vi "PH_AxisGUI_6P.PC AbsMove.vi"(0 "i ref in":refnum<vi>, 2 "Axis Selector":T1, 4 "absolute position (units)":dbl, 5 "error in":errorcluster) -> (14 "i ref out":refnum<vi>, 19 "error out":errorcluster)   [LabVIEW 2014]
uses:
  PH_AxisGUI_6P.lvlib
  PH_Common/PH_Motion/PH_Motion.Axis Address.ctl
  PH_AxisGUI_6P.AxisSelector.ctl
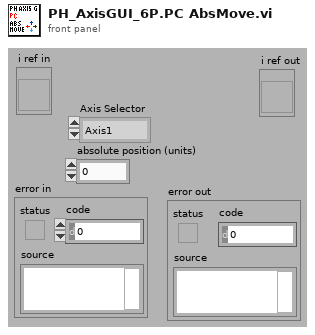
[diagram p1: front panel]
types:
  T1 = typedef "PH_AxisGUI_6P.lvlib/PH_AxisGUI_6P.AxisSelector.ctl" = enum16{"Axis1", "Axis2", "None"}
  T2 = typedef "PH_AxisGUI_6P.lvlib/PH_AxisGUI_6P.i attribute.ctl" = cluster{"GUI Refs":cluster{"AxisSelection":refnum<vi>, "Tab Control":refnum<vi>}}
  T3 = typedef "PH_Motion.Axis Address.ctl" = cluster{"Instance":string, "Motor Nr":i32}
  T4 = typedef "PH_AxisGUI_BaseClass.lvlib/PH_AxisGUI_BaseClass.Dataset In Constructor.ctl" = cluster{"Address":T3, "Name":string, "Label \"Back\"":string, "Labell \"Forth\"":string}
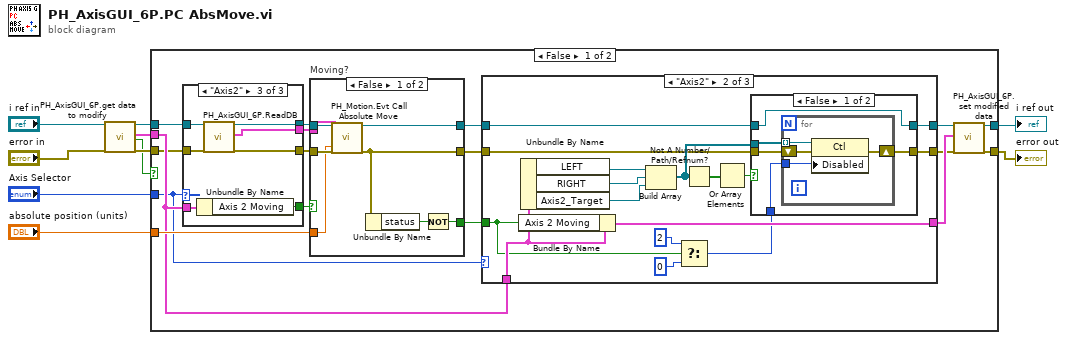
[diagram p0: block diagram]
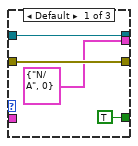
[diagram p2: hidden frame]
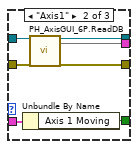
[diagram p3: hidden frame]
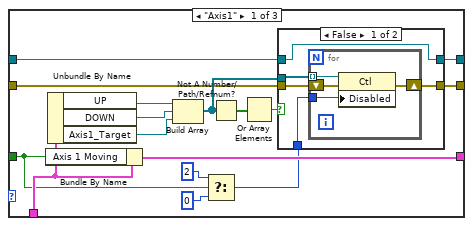
[diagram p4: hidden frame]
diagram:
  n1 = call "PH_AxisGUI_6P.get data to modify.vi"("i ref in"="i ref in", "error in (no error)"="error in") -> ("i ref out"=w4:refnum<vi>, "i attribute"=w1:T2, "timed out"=w2:bool, "error out"=w3:errorcluster)  [unwired: 14 in]
  n2 = case shown="False" w2 {
    tunnel: "Axis Selector" -> [w17 _]
    tunnel: "absolute position (units)" -> [w27 _]
    tunnel: [w26 w115] -> w6
    tunnel: [w25 w114] -> w5
    tunnel: w4 -> [w15 w115]
    tunnel: w3 -> [w14 w114]
    tunnel: w1 -> [w18 _]
    frame False {
      n3 = case shown="\"Axis2\"" w17 {
        tunnel: w18 -> [_ w38 w45]
        tunnel: [TRUE ("Moving") w37 w44] -> w16
        tunnel: w15 -> [w31 w36 w43]
        tunnel: w14 -> [w30 w35 w42]
        tunnel: [w31 w34 w41] -> w13
        tunnel: [w30 w33 w40] -> w12
        tunnel: [T3 {"Instance"="N/A", "Motor Nr"=0} ("Address Axis 2") w32 w39] -> w11
        frame Default {
        }
        frame "Axis1" {
          n4 = Unbundle By Name(w38) -> ("Axis 1 Moving"=w37:bool)
          n5 = call "PH_AxisGUI_6P.ReadDB.vi"("i ref in"=w36, "error in (no error)"=w35) -> ("i ref out"=w34:refnum<vi>, 15:w32, "error out"=w33:errorcluster)  [unwired: 14 in, 1 out]
        }
        frame "Axis2" {
          n6 = Unbundle By Name(w45) -> ("Axis 2 Moving"=w44:bool)
          n7 = call "PH_AxisGUI_6P.ReadDB.vi"("i ref in"=w43, "error in (no error)"=w42) -> ("i ref out"=w41:refnum<vi>, "Data In Base Axis GUI Constructor"=w39:T4[], "error out"=w40:errorcluster)  [unwired: 15 in]
        }
      }
      n8 = case "Moving?" shown="False" w16 {
        selector: w16 -> [_ w111]
        tunnel: w11 -> [w110 _]
        tunnel: w13 -> [w109 w113]
        tunnel: [w108 w113] -> w24
        tunnel: [w105 w112] -> w23
        tunnel: w12 -> [w107 w112]
        tunnel: w27 -> [w106 _]
        tunnel: [w104 w111] -> w22
        frame False {
          n9 = call "PH_Motion.Evt Call Absolute Move.vi"("i ref in"=w109, "Address"=w110, "error in"=w107, "Target Position (Units)"=w106) -> ("i ref out"=w108:refnum<vi>, "error out"=w105:errorcluster)  [unwired: 14 in]
          n10 = Unbundle By Name(w105) -> ("status"=w103:bool)
          n11 = Not(x=w103) -> (.not. x?=w104:bool)
        }
        frame True {
        }
      }
      n12 = case shown="\"Axis2\"" w17 {
        tunnel: w18 -> [w60 w87 w102]
        tunnel: [w61 w88 w102] -> w21
        tunnel: w22 -> [w48 w75 _]
        tunnel: [w53 w80 w100] -> w20
        tunnel: [w52 w79 w101] -> w19
        tunnel: w24 -> [w51 w78 w101]
        tunnel: w23 -> [w50 w77 w100]
        frame "Axis1" {
          n13 = Bundle By Name(cluster=w60, "Axis 1 Moving"=w48) -> (w61:T2)
          n14 = Unbundle By Name(w60) -> ("UP"=w59:refnum<vi>, "DOWN"=w58:refnum<vi>, "Axis1_Target"=w57:refnum<vi>)
          n15 = Build Array(w59, w58, w57) -> (w54:refnum<vi>[])
          n16 = Select(t=u8 2 ("Disabled"), s=w48, f=u8 0 ("Disabled")) -> (s? t:f=w49:u8)
          n17 = Not A Number/Path/Refnum?(number/path/refnum=w54) -> (NaN/Path/Refnum?=w56:bool[])
          n18 = Or Array Elements(Boolean array=w56) -> (logical OR=w55:bool)
          n19 = case shown="False" w55 {
            tunnel: w54 -> [w63 _]
            tunnel: [w66 w71] -> w53
            tunnel: [w65 w72] -> w52
            tunnel: w51 -> [w65 w72]
            tunnel: w50 -> [w64 w71]
            tunnel: w49 -> [w62 _]
            frame False {
              n20 = for {
                shift-right: [w69] -> w66
                shift-left: w64 -> [w70]
                tunnel: w63 -> [w68] mode=indexing
                tunnel: w62 -> [w67]
                n21 = property class="Ctl"(reference=w68, error in=w70, "Disabled"=w67) -> (error out=w69:errorcluster)  [unwired: 1 out]
              }
            }
            frame True {
            }
          }
        }
        frame "Axis2" {
          n22 = Bundle By Name(cluster=w87, "Axis 2 Moving"=w75) -> (w88:T2)
          n23 = Unbundle By Name(w87) -> ("LEFT"=w86:refnum<vi>, "RIGHT"=w85:refnum<vi>, "Axis2_Target"=w84:refnum<vi>)
          n24 = Build Array(w86, w85, w84) -> (w81:refnum<vi>[])
          n25 = Select(t=u8 2 ("Disabled"), s=w75, f=u8 0 ("Disabled")) -> (s? t:f=w76:u8)
          n26 = Not A Number/Path/Refnum?(number/path/refnum=w81) -> (NaN/Path/Refnum?=w83:bool[])
          n27 = Or Array Elements(Boolean array=w83) -> (logical OR=w82:bool)
          n28 = case shown="False" w82 {
            tunnel: w81 -> [w90 _]
            tunnel: [w93 w98] -> w80
            tunnel: [w92 w99] -> w79
            tunnel: w78 -> [w92 w99]
            tunnel: w77 -> [w91 w98]
            tunnel: w76 -> [w89 _]
            frame False {
              n29 = for {
                shift-right: [w96] -> w93
                shift-left: w91 -> [w97]
                tunnel: w90 -> [w95] mode=indexing
                tunnel: w89 -> [w94]
                n30 = property class="Ctl"(reference=w95, error in=w97, "Disabled"=w94) -> (error out=w96:errorcluster)  [unwired: 1 out]
              }
            }
            frame True {
            }
          }
        }
        frame "None", Default {
        }
      }
      n31 = call "PH_AxisGUI_6P.set modified data.vi"("i ref in"=w19, "i attribute"=w21, "error in (no error)"=w20) -> ("i ref out"=w26:refnum<vi>, "error out"=w25:errorcluster)  [unwired: 15 in]
    }
    frame True {
    }
  }
  "error out" <- w5
  "i ref out" <- w6
